vi "Configure Modulation Low Level (Function).vi"(8 "error in (no error)":errorcluster, 9 "Function (Sine)":T1(ring), 10 "Modulation (AM)":enum16{"AM", "FM", "PM", "PWM"}(ring), 11 "VISA resource name":refnum<visa-resource-name>) -> (0 "error out":errorcluster, 3 "VISA resource name out":refnum<visa-resource-name>)   [LabVIEW 2017, in "Keithley 3390.lvlib"]
uses:
  Keithley 3390.lvlib
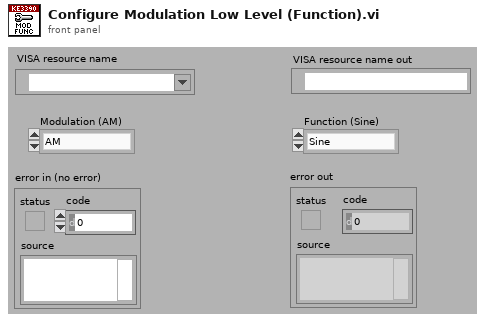
[diagram p1: front panel]
types:
  T1 = enum16{"Sine", "Square", "Ramp", "Negative Ramp", "Triangle", "Noise", "Arbitrary"}
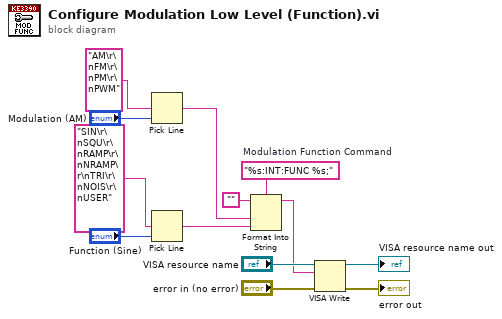
[diagram p0: block diagram]
diagram:
  w7 = "%s:INT:FUNC %s;"  # Modulation Function Command
  n1 = Pick Line(multi-line string="AM\r\nFM\r\nPM\r\nPWM" ("options"), line index="Modulation (AM)") -> (output string=w5:string)  [unwired: 1 in]
  n2 = Pick Line(multi-line string="SIN\r\nSQU\r\nRAMP\r\nNRAMP\r\nTRI\r\nNOIS\r\nUSER" ("options"), line index="Function (Sine)") -> (output string=w6:string)  [unwired: 1 in]
  n3 = Format Into String(format string=w7, initial string="", w5, w6) -> (resulting string=w3:string)  [unwired: 1 in, 1 out]
  n4 = VISA Write(VISA resource name="VISA resource name", write buffer=w3, error in (no error)="error in (no error)") -> (VISA resource name out=→"VISA resource name out":refnum<visa-resource-name>, error out=→"error out":errorcluster)  [unwired: 1 out]
